vi "Read Record Data.vi"(8 "Error In (no error)":errorcluster, 11 "Expenses Tracker Cycle In":refnum<class "Expenses Tracker Cycle.lvclass">) -> (0 "Error Out":errorcluster, 2 "Record":variant, 3 "Expenses Tracker Cycle Out":refnum<class "Expenses Tracker Cycle.lvclass">)   [LabVIEW 2023, in "Expenses Tracker Cycle.lvclass"]
uses:
  Expenses Tracker Cycle.lvclass
  Expenses Tracker Cycle.lvclass/Expenses Tracker Cycle.ctl
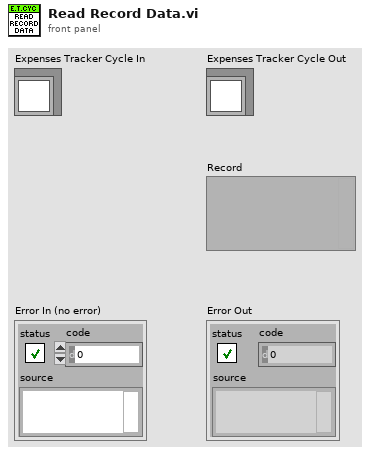
[diagram p1: front panel]
types:
  T1 = typedef "Expenses Tracker Cycle.lvclass/Cycle.ctl" = cluster{"ID":u32, "Name":string, "Day_of_occurence":u8, "Description":string}
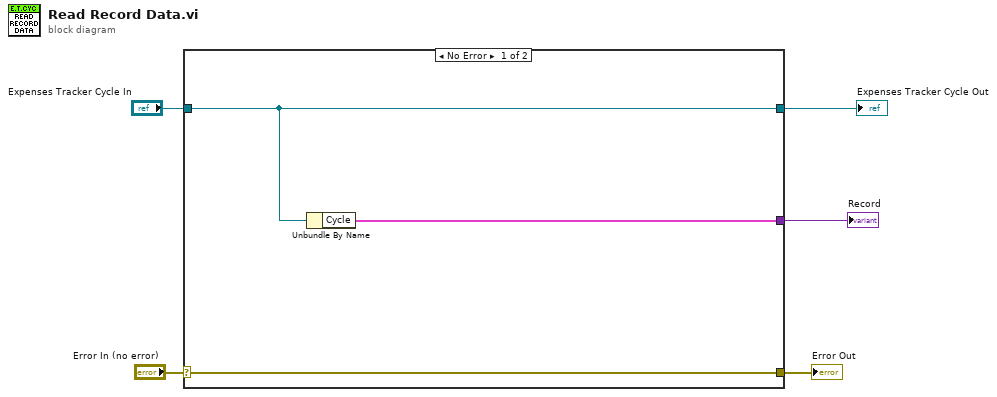
[diagram p0: block diagram]
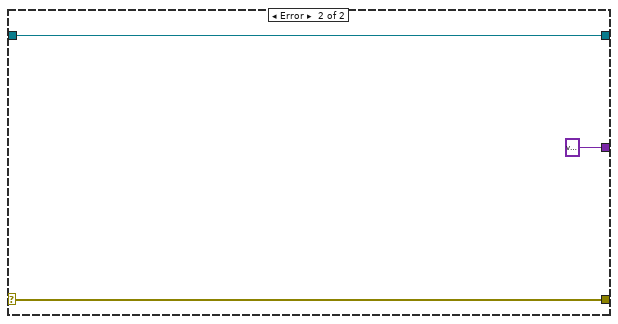
[diagram p2: hidden frame]
diagram:
  n1 = case shown="No Error" "Error In (no error)" {
    selector: "Error In (no error)" -> [w8 w11]
    tunnel: [w8 w11] -> w2
    tunnel: [w7 w10] -> w5
    tunnel: "Expenses Tracker Cycle In" -> [w7 w10]
    tunnel: [w6 variant] -> w1
    frame No Error {
      n2 = Unbundle By Name(w7) -> ("Cycle"=w6:T1)
    }
    frame Error {
    }
  }
  "Error Out" <- w2
  "Expenses Tracker Cycle Out" <- w5
  "Record" <- w1
